vi "sql-delete.vi"(0 "input-IP":string="sql2012agl01.luxshare.com.cn", 1 "input-user":string="htpsuser\n", 2 "input-psw":string="htps'songyy", 3 "input-db":string="HTPSDB", 4 "操作模式":T2(ring)=enum."删除数据", 5 "列名":string[](array[string]), 6 "表名":string="vproject", 7 "数据类型":string[](array[combo]), 8 "DBSet":T1, 9 "主键":string, 11 "限定条件":string) -> (12 "错误类型":string, 15 "status":bool)   [LabVIEW 2011]
panel:
  out "字符串":string
  out "错误输出 1":errorcluster
  out "code":i32
  out "错误输出":errorcluster
  in  "ADODB._Recordset":refnum<k7>
  in  "ADODB._Connection":refnum<k7>
  # "输       入"
  # "输       出"
  # "基本信息\n（）"
  # "创建表、添加表列、删除表列时需要填写\n\n创建的表的列名称、添加的列的名称、删除的列的名称\n\n后面的数据类型，为创建表、添加列时才需要指定的，定义列的数据类型"
  # "状态灯，False表示操作失败，True表示操作成功"
  # "错误类型"
  # "改变操作时需要修改的信息"
  # "操作模式：创建表\n                  删除表\n                  添加表列\n                  删除表列"
  # "表名"
  # "主键，只有在创建表的时候才需要填写，指定创建表列中的一列为主键"
  # "创建表、添加表列、删除表列时需要选择\n\n创建的表所包含的列数、添加的列数、删除的列数"
  # "删除用户时需要填写，利用条件查找需要删除的用户行"
  # "error:\n-2147217843 登陆失败： 。\n-2147467259 要访问的数据库不存在\n-2146825267 没有数据    。\n-2146824584 对象关闭时，不允许操作\n-2147217865 表名不存在 。\n-2147467259 服务器连接失败 。"
  # "error:\n-2147217900 所创建的表已经存在\n-2147217900 该列不存在"
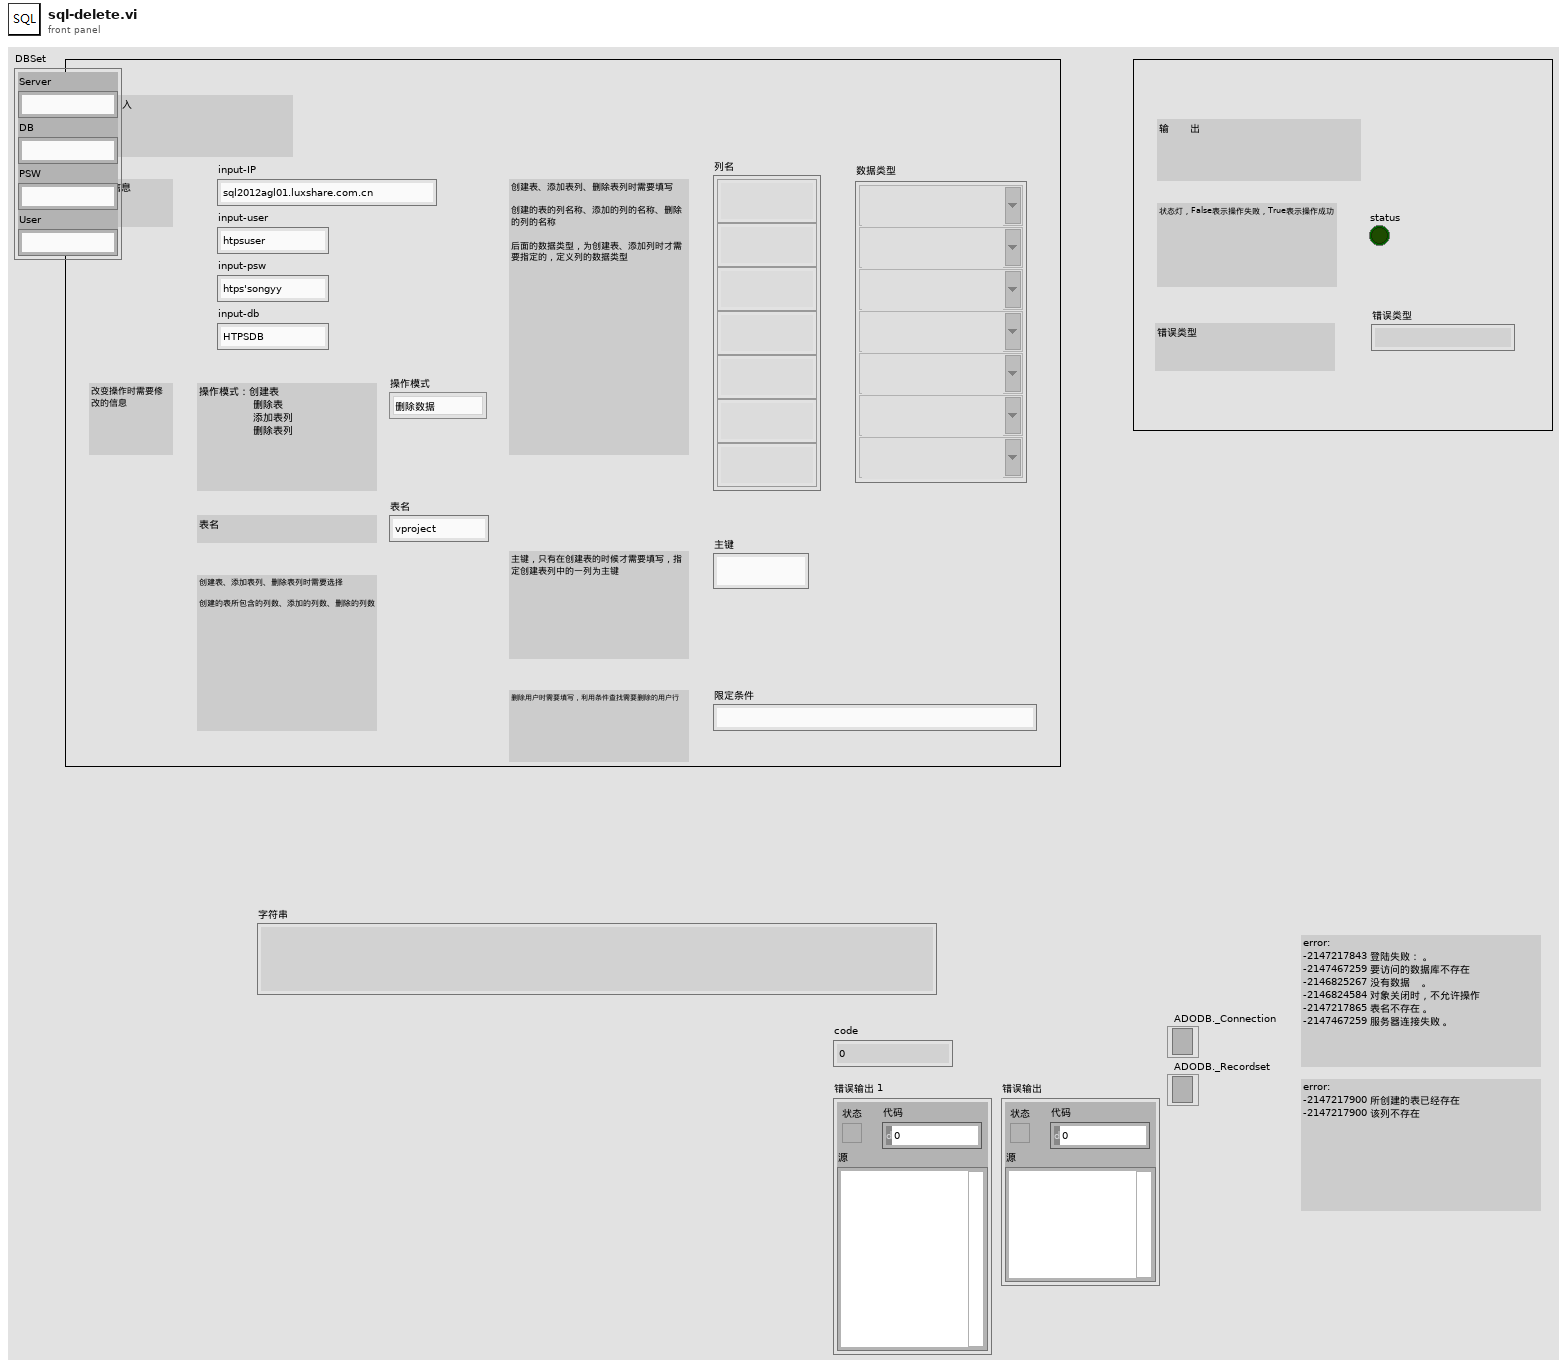
[diagram p1: front panel]
types:
  T1 = cluster{"Server":string, "DB":string, "PSW":string, "User":string}
  T2 = enum16{"", "创建表", "删除表", "添加表列", "删除表列", "添加数据", "删除数据"}
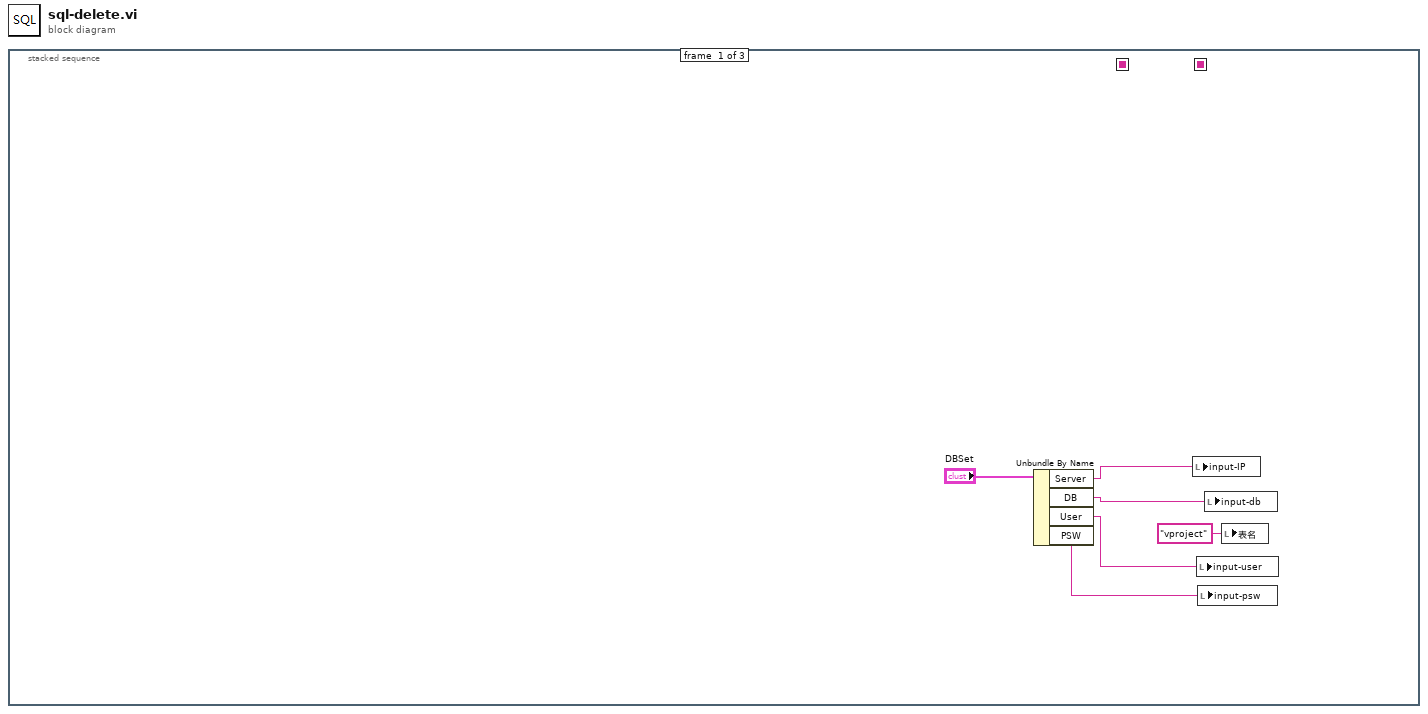
[diagram p0: block diagram]
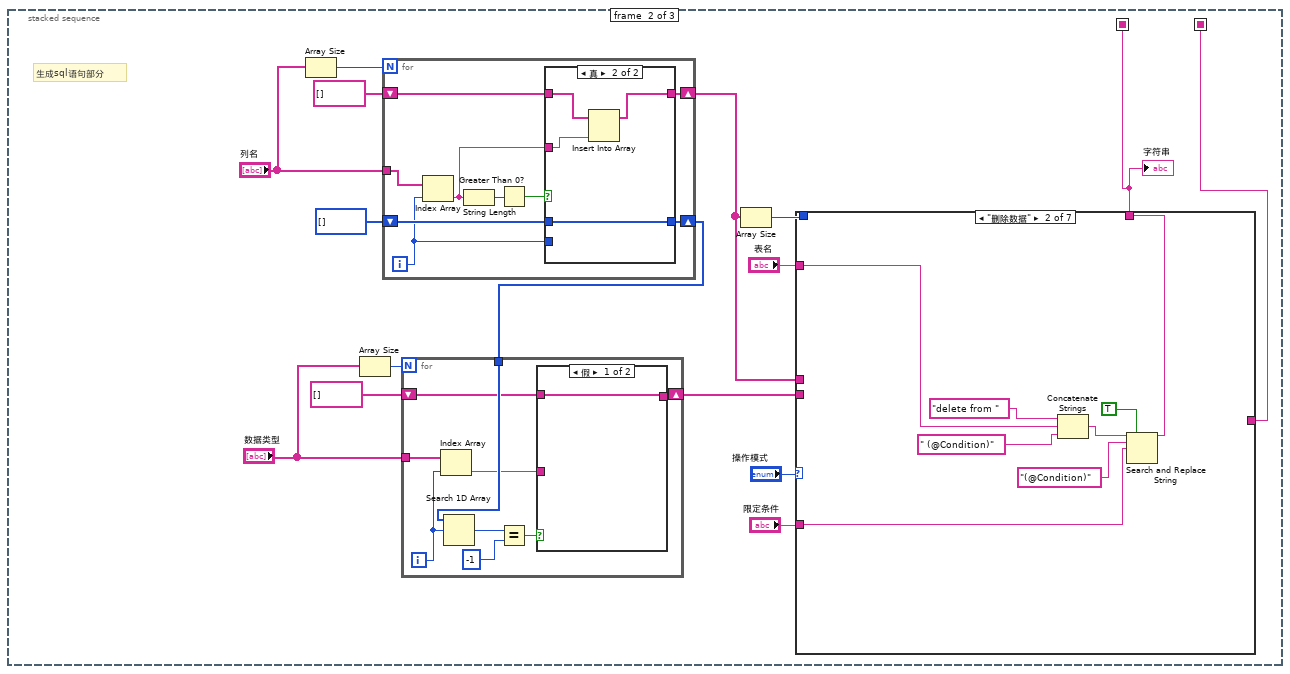
[diagram p2: hidden frame]
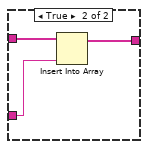
[diagram p3: hidden frame]
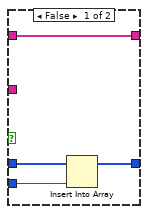
[diagram p4: hidden frame]
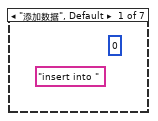
[diagram p5: hidden frame]
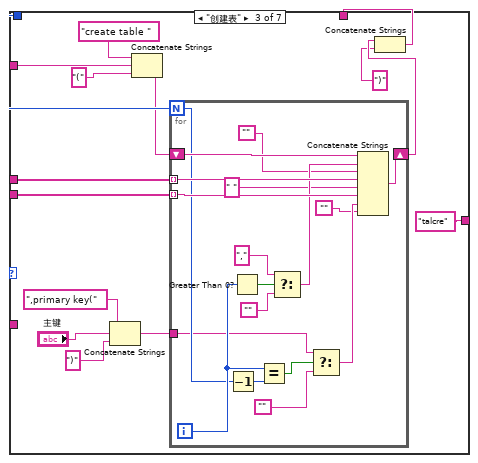
[diagram p6: hidden frame]
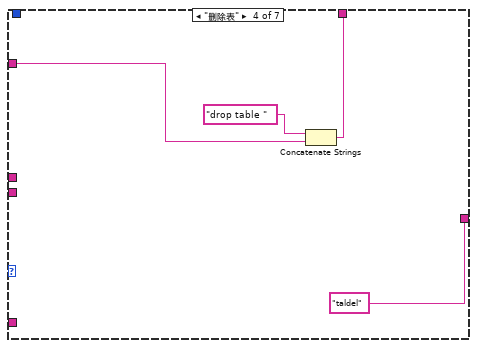
[diagram p7: hidden frame]
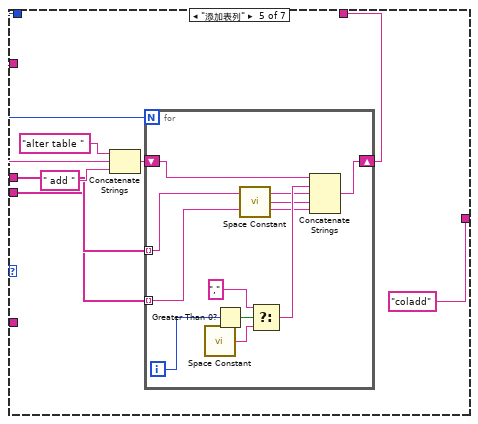
[diagram p8: hidden frame]
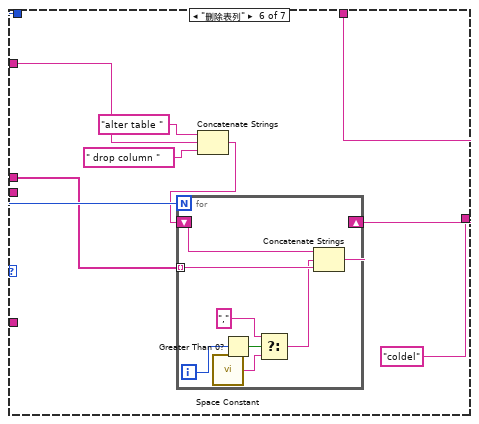
[diagram p9: hidden frame]
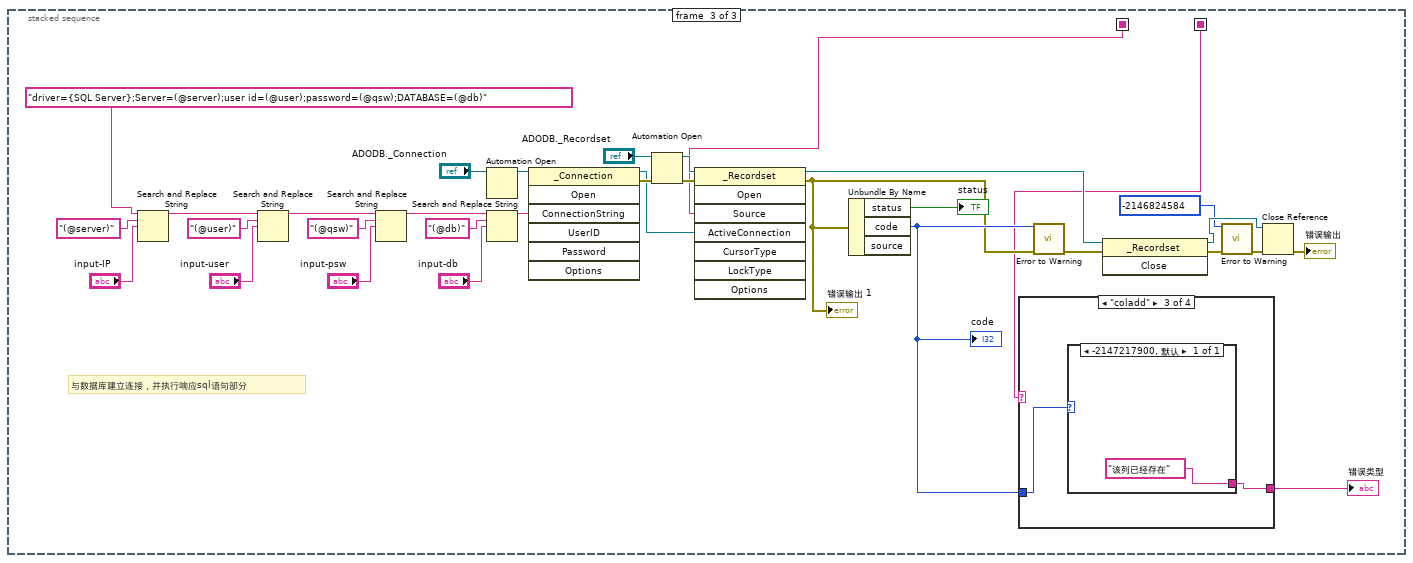
[diagram p11: hidden frame]
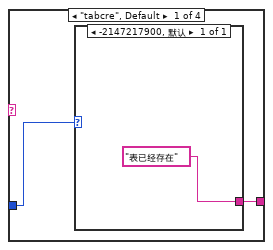
[diagram p12: hidden frame]
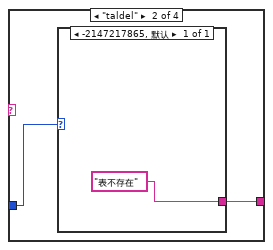
[diagram p13: hidden frame]
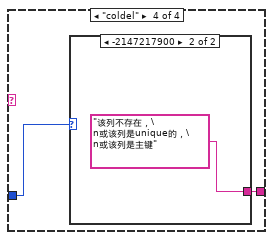
[diagram p14: hidden frame]
diagram:
  n1 = stacked-sequence {
    seq-local: [_ w7 _] -> [_ _ w135]
    seq-local: [_ w8 _] -> [_ _ w134]
    frame #0 {
      n2 = Unbundle By Name("DBSet") -> ("Server"=w5:string, "DB"=w4:string, "User"=w3:string, "PSW"=w2:string)
      n3 = local write "input-IP"(w5) -> ()
      n4 = local write "input-user"(w3) -> ()
      n5 = local write "input-psw"(w2) -> ()
      n6 = local write "input-db"(w4) -> ()
      n7 = local write "表名"("vproject" ("表名")) -> ()
    }
    frame #1 {
      # "生成sql语句部分"
      n8 = Array Size(array="列名") -> (size(s)=w20:i32)
      n9 = Array Size(array="数据类型") -> (size(s)=w17:i32)
      n10 = for {
        N: w20 -> [_]
        tunnel: "列名" -> [w44]
        shift-right: [w39] -> w11
        shift-left: string[] [] -> [w40]
        shift-right: [w36] -> w15
        shift-left: i32[] [] -> [w38]
        i -> [w37]
        n11 = Index Array(array=w44, index=w37) -> (element=w41:string)
        n12 = String Length(string=w41) -> (length=w43:i32)
        n13 = Greater Than 0?(x=w43) -> (x > 0?=w42:bool)
        n14 = case shown="真" w42 {
          tunnel: w41 -> [_ w50]
          tunnel: w40 -> [w48 w52]
          tunnel: [w48 w51] -> w39
          tunnel: w38 -> [w47 w49]
          tunnel: w37 -> [w46 _]
          tunnel: [w45 w49] -> w36
          frame False {
            n15 = Insert Into Array(array=w47, new element=w46) -> (w45:i32[])  [unwired: 1 in]
          }
          frame True {
            n16 = Insert Into Array(array=w52, new element=w50) -> (w51:string[])  [unwired: 1 in]
          }
        }
      }
      n17 = for {
        N: w17 -> [_]
        shift-right: [w23] -> w9
        shift-left: string[] [] -> [w24]
        tunnel: "数据类型" -> [w28]
        tunnel: w15 -> [w31]
        i -> [w27]
        n18 = Index Array(array=w28, index=w27) -> (element=w25:string)
        n19 = Search 1D Array(1D array=w31, element=w27) -> (index of element=w30:i32)  [unwired: 1 in]
        n20 = Equal?(x=w30, y=-1) -> (x = y?=w26:bool)
        n21 = case shown="假" w26 {
          tunnel: w25 -> [_ w33]
          tunnel: w24 -> [w32 w35]
          tunnel: [w32 w34] -> w23
          frame False {
          }
          frame True {
            n22 = Insert Into Array(array=w35, new element=w33) -> (w34:string[])  [unwired: 1 in]
          }
        }
      }
      n23 = Array Size(array=w11) -> (size(s)=w12:i32)
      n24 = case shown="\"删除数据\"" "操作模式" {
        tunnel: "表名" -> [_ w59 w73 w96 w104 w123 _]
        tunnel: [_ w56 w61 w95 w99 w118 _] -> w7
        tunnel: w12 -> [_ _ w75 _ w105 w121 _]
        tunnel: w11 -> [_ _ w62 _ w102 w119 _]
        tunnel: w9 -> [_ _ w71 _ w98 _ _]
        tunnel: [_ _ "talcre" "taldel" "coladd" "coldel" _] -> w8
        tunnel: "限定条件" -> [_ w53 _ _ _ _ _]
        frame "添加数据", Default {
          (unwired) "insert into "
          (unwired) 0
        }
        frame "删除数据" {
          n25 = Concatenate Strings("delete from ", w59, " (@Condition)") -> (w57:string)
          n26 = Search and Replace String(replace all?=TRUE ("替换全部？(F)"), input string=w57, search string="(@Condition)" ("搜索字符串"), replace string=w53) -> (result string=w56:string)  [unwired: 4 in, 3 out]
        }
        frame "创建表" {
          n27 = Concatenate Strings(",primary key(", "主键", ")") -> (w66:string)
          n28 = Concatenate Strings("create table ", w73, "(" ("字符串")) -> (w70:string)
          n29 = for {
            N: w75 -> [w84]
            tunnel: w62 -> [w93] mode=indexing
            tunnel: w71 -> [w92] mode=indexing
            shift-right: [w79] -> w65
            shift-left: w70 -> [w88]
            tunnel: w66 -> [w82]
            i -> [w86]
            n30 = Decrement(x=w84) -> (x-1=w85:i32)
            n31 = Greater Than 0?(x=w86) -> (x > 0?=w91:bool)
            n32 = Equal?(x=w86, y=w85) -> (x = y?=w83:bool)
            n33 = Select(t=",", s=w91, f="") -> (s? t:f=w87:string)
            n34 = Select(t=w82, s=w83, f="") -> (s? t:f=w80:string)
            n35 = Concatenate Strings(w88, w87, "", w93, " ", w92, w80, "") -> (w79:string)
          }
          n36 = Concatenate Strings(w65, ")") -> (w61:string)
        }
        frame "删除表" {
          n37 = Concatenate Strings("drop table ", w96) -> (w95:string)
        }
        frame "添加表列" {
          n38 = Concatenate Strings("alter table ", w104, " add ") -> (w101:string)
          n39 = for {
            N: w105 -> [_]
            tunnel: w102 -> [w110] mode=indexing
            shift-right: [w109] -> w99
            shift-left: w101 -> [w116]
            tunnel: w98 -> [w108] mode=indexing
            i -> [w112]
            n40 = call <vilib>:"Space Constant.vi"() -> ("String"=w113:string)
            n41 = Greater Than 0?(x=w112) -> (x > 0?=w115:bool)
            n42 = call <vilib>:"Space Constant.vi"() -> ("String"=w107:string)
            n43 = Select(t=",", s=w115, f=w113) -> (s? t:f=w111:string)
            n44 = Concatenate Strings(w116, w111, w110, w107, w108) -> (w109:string)
          }
        }
        frame "删除表列" {
          n45 = Concatenate Strings("alter table ", w123, " drop column ") -> (w120:string)
          n46 = for {
            N: w121 -> [_]
            tunnel: w119 -> [w131] mode=indexing
            shift-right: [w125] -> w118
            shift-left: w120 -> [w132]
            i -> [w126]
            n47 = call <vilib>:"Space Constant.vi"() -> ("String"=w130:string)
            n48 = Greater Than 0?(x=w126) -> (x > 0?=w128:bool)
            n49 = Select(t=",", s=w128, f=w130) -> (s? t:f=w127:string)
            n50 = Concatenate Strings(w132, w127, w131) -> (w125:string)
          }
        }
        frame "" {
        }
      }
      "字符串" <- w7
    }
    frame #2 {
      # "与数据库建立连接，并执行响应sql语句部分"
      n51 = Search and Replace String(input string="driver={SQL Server};Server=(@server);user id=(@user);password=(@qsw);DATABASE=(@db)" ("ConnectionString"), search string="(@server)" ("搜索字符串"), replace string="input-IP") -> (result string=w140:string)  [unwired: 5 in, 3 out]
      n52 = Search and Replace String(input string=w140, search string="(@user)" ("搜索字符串"), replace string="input-user") -> (result string=w143:string)  [unwired: 5 in, 3 out]
      n53 = Search and Replace String(input string=w143, search string="(@qsw)" ("搜索字符串"), replace string="input-psw") -> (result string=w146:string)  [unwired: 5 in, 3 out]
      n54 = Automation Open(Automation Refnum="ADODB._Connection") -> (Automation Refnum=w136:refnum<k7>)  [unwired: 3 in, 1 out]
      n55 = Search and Replace String(input string=w146, search string="(@db)" ("搜索字符串"), replace string="input-db") -> (result string=w150:string)  [unwired: 5 in, 3 out]
      n56 = invoke class="_Connection" method="Open"(reference=w136, "ConnectionString"=w150) -> (reference out=w152:refnum<k7>, error out=w154:errorcluster)  [unwired: 5 in, 5 out]
      n57 = Automation Open(error in (no error)=w154, Automation Refnum="ADODB._Recordset") -> (Automation Refnum=w153:refnum<k7>, error out=w155:errorcluster)  [unwired: 2 in]
      n58 = invoke class="_Recordset" method="Open"(reference=w153, error in=w155, "Source"=w135, "ActiveConnection"=w152) -> (reference out=w162:refnum<k7>, error out=w163:errorcluster)  [unwired: 4 in, 6 out]
      "错误输出 1" <- w163
      n59 = Unbundle By Name(w163) -> ("status"=→"status":bool, "code"=w165:i32)  [unwired: 1 out]
      "code" <- w165
      n60 = case shown="\"coladd\"" w134 {
        tunnel: w165 -> [w167 w170 w173 w176]
        tunnel: [w166 w169 w172 w175] -> w164
        frame "tabcre", Default {
          n61 = case shown="-2147217900, 默认" w167 {
            tunnel: ["表已经存在"] -> w166
            frame -2147217900, Default {
            }
          }
        }
        frame "taldel" {
          n62 = case shown="-2147217865, 默认" w170 {
            tunnel: ["表不存在"] -> w169
            frame -2147217865, Default {
            }
          }
        }
        frame "coladd" {
          n63 = case shown="-2147217900, 默认" w173 {
            tunnel: ["该列已经存在"] -> w172
            frame -2147217900, Default {
            }
          }
        }
        frame "coldel" {
          n64 = case shown="-2147217900" w176 {
            tunnel: [_ "该列不存在，\n或该列是unique的，\n或该列是主键"] -> w175
            frame 0, Default {
            }
            frame -2147217900 {
            }
          }
        }
      }
      "错误类型" <- w164
      n65 = call <vilib>:"Error to Warning.vi"("1st Error to Convert"=w165, "error in"=w163) -> ("warning out"=w156:errorcluster)  [unwired: 13 in]
      n66 = invoke class="_Recordset" method="Close"(reference=w162, error in=w156) -> (reference out=w160:refnum<k7>, error out=w157:errorcluster)  [unwired: 1 in, 1 out]
      n67 = call <vilib>:"Error to Warning.vi"("1st Error to Convert"=-2146824584, "error in"=w157) -> ("warning out"=w161:errorcluster)  [unwired: 13 in]
      n68 = Close Reference(reference=w160, error in (no error)=w161) -> (error out=→"错误输出":errorcluster)
    }
  }
